vi "Initialize RF boards - with FPGA init only vi 16.3.1v7d.vi"(2 "error in":errorcluster, 3 "FPGA Interface":T1) -> (0 "error out":errorcluster, 1 "FPGA Interface 2":T1)   [LabVIEW 2012]
uses:
  openfpgaref.initrf.ctl
  <vilib>/Utility/error.llb/Error Cluster From Error Code.vi
  <vilib>/rvi/errors/niLvFpgaAdjustHostInterfaceError.vi
  <vilib>/rvi/interface/nirviReadWriteControl/nirviReadWriteControl.xnode
  FPGA Bitfiles/UHR-FleezersInst_FPGATarget_intitializeRFsyn_v1.lvbitx
  NiFpgaLv.dll
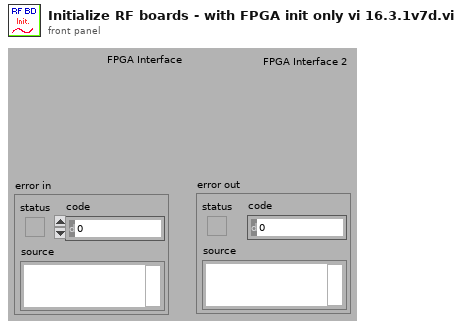
[diagram p1: front panel]
types:
  T1 = typedef "openfpgaref.initrf.ctl" = refnum<k20>
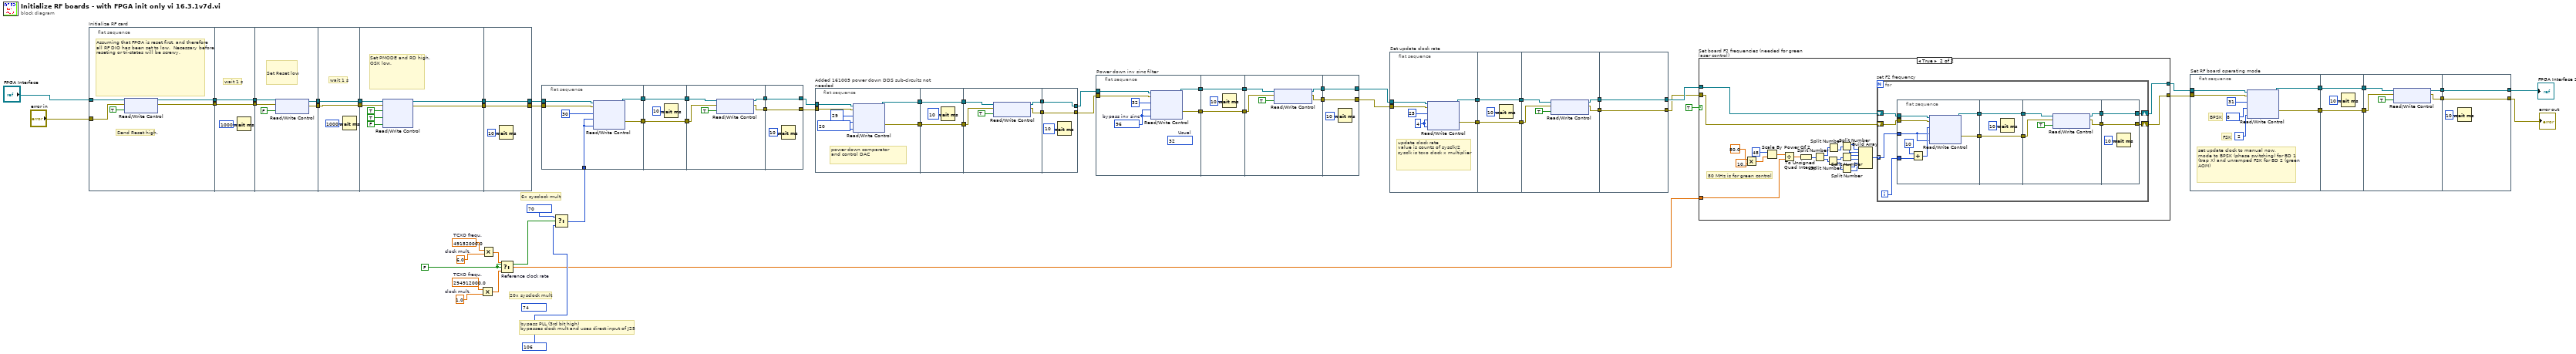
[diagram p0: block diagram]
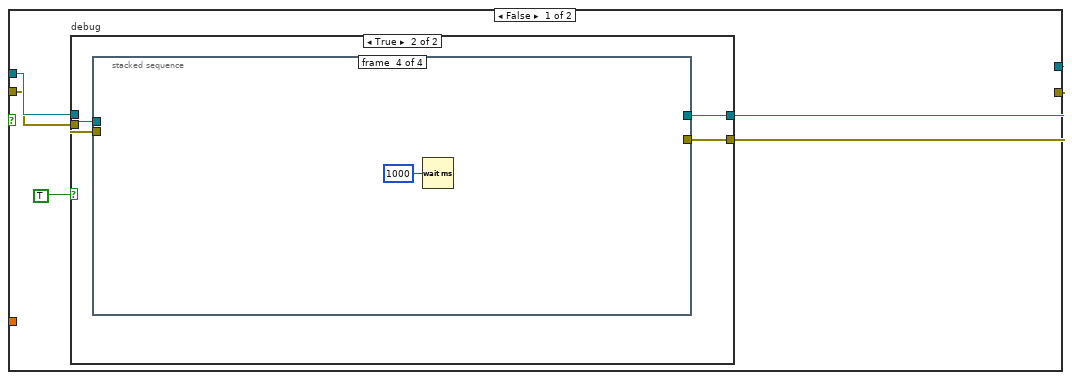
[diagram p2: hidden frame]
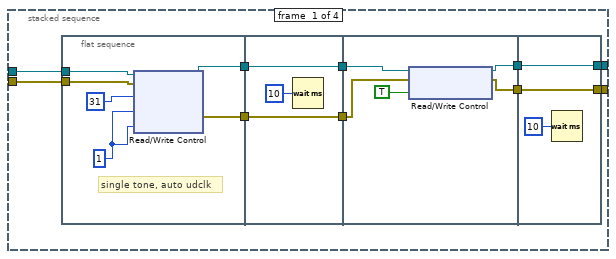
[diagram p4: hidden frame]
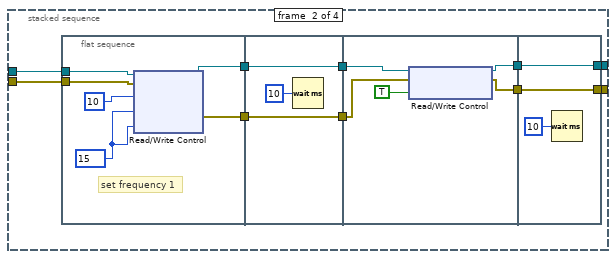
[diagram p5: hidden frame]
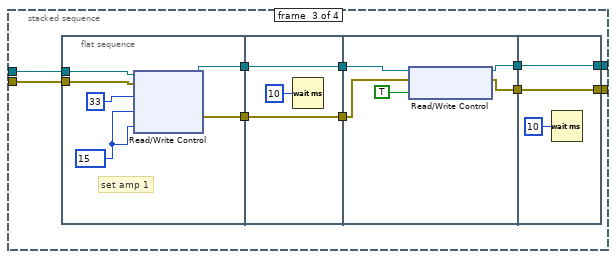
[diagram p6: hidden frame]
diagram:
  (unwired) u8 74 ("Data")
  w19 = FALSE ("s")
  w22 = 1.0  # clock mult.
  w21 = 294912000.0  # TCXO frequ.
  w25 = 6.0  # clock mult.
  w24 = 49152000.0  # TCXO frequ.
  # "bypass PLL (3rd bit high)\nbypasses clock mult and uses direct input of J25"
  # "20x sysclock mult"
  # "6x sysclock mult"
  n1 = flat-sequence "Initialize RF card" {
    tunnel: [w73] -> w68
    tunnel: [w72] -> w67
    tunnel: "error in" -> [w71]
    tunnel: "FPGA Interface" -> [w69]
    tunnel: w68 -> [w75]
    tunnel: w67 -> [w74]
    tunnel: [w75] -> w66
    tunnel: [w74] -> w65
    tunnel: w66 -> [w81]
    tunnel: w65 -> [w80]
    tunnel: [w79] -> w64
    tunnel: [w78] -> w63
    tunnel: w64 -> [w83]
    tunnel: w63 -> [w82]
    tunnel: [w83] -> w62
    tunnel: [w82] -> w61
    tunnel: w62 -> [w91]
    tunnel: w61 -> [w90]
    tunnel: [w87] -> w51
    tunnel: [w86] -> w50
    tunnel: [w93] -> w44
    tunnel: [w94] -> w45
    tunnel: w51 -> [w94]
    tunnel: w50 -> [w93]
    frame #0 {
      # "Send Reset high."
      # "Assuming that FPGA is reset first, and therefore\nall RF DIO has been set to low.  Necessary before\nreseting or tri-states will be screwy."
      n2 = xnode "Read/Write Control"("FPGA VI Reference In"=w69, "error in"=w71, "Reset Bd 1"=TRUE ("Reset")) -> ("FPGA VI Reference Out"=w73:T1, "error out"=w72:errorcluster)
    }
    frame #1 {
      # "wait 1 s"
      n3 = Wait (ms)(milliseconds to wait=u32 1000) -> ()  [unwired: 1 out]
    }
    frame #2 {
      # "Set Reset low"
      n4 = xnode "Read/Write Control"("FPGA VI Reference In"=w81, "error in"=w80, "Reset Bd 1"=FALSE ("Reset")) -> ("FPGA VI Reference Out"=w79:T1, "error out"=w78:errorcluster)
    }
    frame #3 {
      # "wait 1 s"
      n5 = Wait (ms)(milliseconds to wait=u32 1000) -> ()  [unwired: 1 out]
    }
    frame #4 {
      # "Set PMODE and RD high,\nOSK low."
      n6 = xnode "Read/Write Control"("FPGA VI Reference In"=w91, "error in"=w90, "RD"=TRUE, "PMODE"=TRUE, "OSK Bd 1"=FALSE ("OSK")) -> ("FPGA VI Reference Out"=w87:T1, "error out"=w86:errorcluster)
    }
    frame #5 {
      n7 = Wait (ms)(milliseconds to wait=u32 10) -> ()  [unwired: 1 out]
    }
  }
  n8 = Multiply(x=w21, y=w22) -> (x*y=w20:dbl)
  n9 = Multiply(x=w24, y=w25) -> (x*y=w23:dbl)
  n10 = Select "Reference clock rate"(t=w23, s=w19, f=w20) -> (s? t:f=w1:dbl)
  n11 = flat-sequence {
    tunnel: [w100] -> w60
    tunnel: [w99] -> w59
    tunnel: w45 -> [w98]
    tunnel: w44 -> [w97]
    tunnel: w17 -> [w95]
    tunnel: [w102] -> w58
    tunnel: w60 -> [w102]
    tunnel: [w101] -> w57
    tunnel: w59 -> [w101]
    tunnel: w58 -> [w108]
    tunnel: w57 -> [w107]
    tunnel: [w105] -> w49
    tunnel: [w104] -> w48
    tunnel: [w110] -> w8
    tunnel: [w111] -> w9
    tunnel: w49 -> [w111]
    tunnel: w48 -> [w110]
    frame #0 {
      n12 = xnode "Read/Write Control"("FPGA VI Reference In"=w98, "error in"=w97, "Address"=u8 30, "Data BD 1"=w95, "Data BD 2"=w95) -> ("FPGA VI Reference Out"=w100:T1, "error out"=w99:errorcluster)
    }
    frame #1 {
      n13 = Wait (ms)(milliseconds to wait=u32 10) -> ()  [unwired: 1 out]
    }
    frame #2 {
      n14 = xnode "Read/Write Control"("FPGA VI Reference In"=w108, "error in"=w107, "Update Data"=TRUE) -> ("FPGA VI Reference Out"=w105:T1, "error out"=w104:errorcluster)
    }
    frame #3 {
      n15 = Wait (ms)(milliseconds to wait=u32 10) -> ()  [unwired: 1 out]
    }
  }
  n16 = Select(t=u8 70 ("Data"), s=w19, f=u8 106 ("Data")) -> (s? t:f=w17:u8)
  n17 = flat-sequence "Added 161005 power down DDS sub-circuits not needed" {
    tunnel: [w117] -> w15
    tunnel: [w116] -> w14
    tunnel: w9 -> [w115]
    tunnel: w8 -> [w114]
    tunnel: [w119] -> w13
    tunnel: w15 -> [w119]
    tunnel: [w118] -> w12
    tunnel: w14 -> [w118]
    tunnel: w13 -> [w125]
    tunnel: w12 -> [w124]
    tunnel: [w122] -> w11
    tunnel: [w121] -> w10
    tunnel: [w128] -> w6
    tunnel: w11 -> [w126]
    tunnel: w10 -> [w128]
    tunnel: [w126] -> w7
    frame #0 {
      w112 = u8 20 ("Data")
      # "power down comparator\nand control DAC"
      n18 = xnode "Read/Write Control"("FPGA VI Reference In"=w115, "error in"=w114, "Address"=u8 29, "Data BD 1"=w112, "Data BD 2"=w112) -> ("FPGA VI Reference Out"=w117:T1, "error out"=w116:errorcluster)
    }
    frame #1 {
      n19 = Wait (ms)(milliseconds to wait=u32 10) -> ()  [unwired: 1 out]
    }
    frame #2 {
      n20 = xnode "Read/Write Control"("FPGA VI Reference In"=w125, "error in"=w124, "Update Data"=TRUE) -> ("FPGA VI Reference Out"=w122:T1, "error out"=w121:errorcluster)
    }
    frame #3 {
      n21 = Wait (ms)(milliseconds to wait=u32 10) -> ()  [unwired: 1 out]
    }
  }
  n22 = flat-sequence "Power down inv sinc filter" {
    tunnel: [w134] -> w56
    tunnel: [w133] -> w55
    tunnel: w7 -> [w132]
    tunnel: w6 -> [w131]
    tunnel: [w136] -> w54
    tunnel: w56 -> [w136]
    tunnel: [w135] -> w53
    tunnel: w55 -> [w135]
    tunnel: w54 -> [w142]
    tunnel: w53 -> [w141]
    tunnel: [w139] -> w47
    tunnel: [w138] -> w46
    tunnel: [w144] -> w36
    tunnel: [w145] -> w37
    tunnel: w47 -> [w145]
    tunnel: w46 -> [w144]
    frame #0 {
      w129 = u8 96  # bypass inv sinc
      (unwired) u8 32  # Usual
      n23 = xnode "Read/Write Control"("FPGA VI Reference In"=w132, "error in"=w131, "Address"=u8 32, "Data BD 1"=w129, "Data BD 2"=w129) -> ("FPGA VI Reference Out"=w134:T1, "error out"=w133:errorcluster)
    }
    frame #1 {
      n24 = Wait (ms)(milliseconds to wait=u32 10) -> ()  [unwired: 1 out]
    }
    frame #2 {
      n25 = xnode "Read/Write Control"("FPGA VI Reference In"=w142, "error in"=w141, "Update Data"=TRUE) -> ("FPGA VI Reference Out"=w139:T1, "error out"=w138:errorcluster)
    }
    frame #3 {
      n26 = Wait (ms)(milliseconds to wait=u32 10) -> ()  [unwired: 1 out]
    }
  }
  n27 = flat-sequence "Set update clock rate" {
    tunnel: [w151] -> w43
    tunnel: [w150] -> w42
    tunnel: w37 -> [w149]
    tunnel: w36 -> [w148]
    tunnel: [w153] -> w41
    tunnel: w43 -> [w153]
    tunnel: [w152] -> w40
    tunnel: w42 -> [w152]
    tunnel: w41 -> [w159]
    tunnel: w40 -> [w158]
    tunnel: [w156] -> w39
    tunnel: [w155] -> w38
    tunnel: [w160] -> w34
    tunnel: [w161] -> w35
    tunnel: w39 -> [w161]
    tunnel: w38 -> [w160]
    frame #0 {
      w146 = u8 4 ("Data")
      # "update clock rate\nvalue is counts of sysclk/2\nsysclk is tcxo clock x multiplier"
      n28 = xnode "Read/Write Control"("FPGA VI Reference In"=w149, "error in"=w148, "Address"=u8 25, "Data BD 1"=w146, "Data BD 2"=w146) -> ("FPGA VI Reference Out"=w151:T1, "error out"=w150:errorcluster)
    }
    frame #1 {
      n29 = Wait (ms)(milliseconds to wait=u32 10) -> ()  [unwired: 1 out]
    }
    frame #2 {
      n30 = xnode "Read/Write Control"("FPGA VI Reference In"=w159, "error in"=w158, "Update Data"=TRUE) -> ("FPGA VI Reference Out"=w156:T1, "error out"=w155:errorcluster)
    }
    frame #3 {
    }
  }
  n31 = case "Set board F2 frequencies (needed for green laser control)" shown="True" TRUE {
    tunnel: w35 -> [w166 w274]
    tunnel: w34 -> [w165 w273]
    tunnel: [w162 w271] -> w33
    tunnel: [w163 w272] -> w32
    tunnel: w1 -> [_ w251]
    frame False {
      n32 = case "debug" shown="True" TRUE {
        tunnel: w166 -> [w168 w172]
        tunnel: w165 -> [w167 w171]
        tunnel: [w168 w170] -> w163
        tunnel: [w167 w169] -> w162
        frame False {
        }
        frame True {
          n33 = stacked-sequence {
            tunnel: w172 -> [w174 w199 w226 _]
            tunnel: w171 -> [w173 w198 w225 _]
            tunnel: [_ _ w224 _] -> w170
            tunnel: [_ _ w223 _] -> w169
            frame #0 {
              n34 = flat-sequence {
                tunnel: [w186] -> w180
                tunnel: [w185] -> w179
                tunnel: w174 -> [w184]
                tunnel: w173 -> [w183]
                tunnel: [w188] -> w178
                tunnel: w180 -> [w188]
                tunnel: [w187] -> w177
                tunnel: w179 -> [w187]
                tunnel: w178 -> [w194]
                tunnel: w177 -> [w193]
                tunnel: [w191] -> w176
                tunnel: [w190] -> w175
                tunnel: [w197] -> _
                tunnel: [w195] -> _
                tunnel: w176 -> [w195]
                tunnel: w175 -> [w197]
                frame #0 {
                  w181 = u8 1 ("Data")
                  # "single tone, auto udclk"
                  n35 = xnode "Read/Write Control"("FPGA VI Reference In"=w184, "error in"=w183, "Address"=u8 31, "Data BD 1"=w181, "Data BD 2"=w181) -> ("FPGA VI Reference Out"=w186:T1, "error out"=w185:errorcluster)
                }
                frame #1 {
                  n36 = Wait (ms)(milliseconds to wait=u32 10) -> ()  [unwired: 1 out]
                }
                frame #2 {
                  n37 = xnode "Read/Write Control"("FPGA VI Reference In"=w194, "error in"=w193, "Update Data"=TRUE) -> ("FPGA VI Reference Out"=w191:T1, "error out"=w190:errorcluster)
                }
                frame #3 {
                  n38 = Wait (ms)(milliseconds to wait=u32 10) -> ()  [unwired: 1 out]
                }
              }
            }
            frame #1 {
              n39 = flat-sequence {
                tunnel: [w211] -> w205
                tunnel: [w210] -> w204
                tunnel: w199 -> [w209]
                tunnel: w198 -> [w208]
                tunnel: [w213] -> w203
                tunnel: w205 -> [w213]
                tunnel: [w212] -> w202
                tunnel: w204 -> [w212]
                tunnel: w203 -> [w219]
                tunnel: w202 -> [w218]
                tunnel: [w216] -> w201
                tunnel: [w215] -> w200
                tunnel: [w222] -> _
                tunnel: [w220] -> _
                tunnel: w201 -> [w220]
                tunnel: w200 -> [w222]
                frame #0 {
                  w206 = u8 15 ("Data")
                  # "set frequency 1"
                  n40 = xnode "Read/Write Control"("FPGA VI Reference In"=w209, "error in"=w208, "Address"=u8 10, "Data BD 1"=w206, "Data BD 2"=w206) -> ("FPGA VI Reference Out"=w211:T1, "error out"=w210:errorcluster)
                }
                frame #1 {
                  n41 = Wait (ms)(milliseconds to wait=u32 10) -> ()  [unwired: 1 out]
                }
                frame #2 {
                  n42 = xnode "Read/Write Control"("FPGA VI Reference In"=w219, "error in"=w218, "Update Data"=TRUE) -> ("FPGA VI Reference Out"=w216:T1, "error out"=w215:errorcluster)
                }
                frame #3 {
                  n43 = Wait (ms)(milliseconds to wait=u32 10) -> ()  [unwired: 1 out]
                }
              }
            }
            frame #2 {
              n44 = flat-sequence {
                tunnel: [w238] -> w232
                tunnel: [w237] -> w231
                tunnel: w226 -> [w236]
                tunnel: w225 -> [w235]
                tunnel: [w240] -> w230
                tunnel: w232 -> [w240]
                tunnel: [w239] -> w229
                tunnel: w231 -> [w239]
                tunnel: w230 -> [w246]
                tunnel: w229 -> [w245]
                tunnel: [w243] -> w228
                tunnel: [w242] -> w227
                tunnel: [w249] -> w223
                tunnel: [w247] -> w224
                tunnel: w228 -> [w247]
                tunnel: w227 -> [w249]
                frame #0 {
                  w233 = u8 15 ("Data")
                  # "set amp 1"
                  n45 = xnode "Read/Write Control"("FPGA VI Reference In"=w236, "error in"=w235, "Address"=u8 33, "Data BD 1"=w233, "Data BD 2"=w233) -> ("FPGA VI Reference Out"=w238:T1, "error out"=w237:errorcluster)
                }
                frame #1 {
                  n46 = Wait (ms)(milliseconds to wait=u32 10) -> ()  [unwired: 1 out]
                }
                frame #2 {
                  n47 = xnode "Read/Write Control"("FPGA VI Reference In"=w246, "error in"=w245, "Update Data"=TRUE) -> ("FPGA VI Reference Out"=w243:T1, "error out"=w242:errorcluster)
                }
                frame #3 {
                  n48 = Wait (ms)(milliseconds to wait=u32 10) -> ()  [unwired: 1 out]
                }
              }
            }
            frame #3 {
              n49 = Wait (ms)(milliseconds to wait=u32 1000) -> ()  [unwired: 1 out]
            }
          }
        }
      }
    }
    frame True {
      # "80 MHz is for green control"
      n50 = Multiply(x=80.0 ("Delta Frequency  (MHz)"), y=1000000.0) -> (x*y=w256:dbl)
      n51 = Scale By Power Of 2(n=48, x=w256) -> (x*2^n=w254:dbl)
      n52 = Divide(x=w254, y=w251) -> (x/y=w255:dbl)
      n53 = To Unsigned Quad Integer(1:w255) -> (0:w259:u64)
      n54 = Split Number(x=w259) -> (hi(x)=w260:u32, lo(x)=w261:u32)
      n55 = Split Number(x=w261) -> (hi(x)=w263:u16, lo(x)=w262:u16)
      n56 = Split Number(x=w260) -> (lo(x)=w264:u16)  [unwired: 1 out]
      n57 = Split Number(x=w264) -> (hi(x)=w265:u8, lo(x)=w266:u8)
      n58 = Split Number(x=w263) -> (hi(x)=w267:u8, lo(x)=w268:u8)
      n59 = Split Number(x=w262) -> (hi(x)=w269:u8, lo(x)=w270:u8)
      n60 = Build Array(w265, w266, w267, w268, w269, w270) -> (w252:u8[])
      n61 = for "set F2 frequency" {
        shift-right: [w277] -> w272
        shift-left: w274 -> [w280]
        shift-right: [w278] -> w271
        shift-left: w273 -> [w279]
        tunnel: w252 -> [w275] mode=indexing
        i -> [w276]
        n62 = flat-sequence {
          tunnel: [w294] -> w286
          tunnel: [w293] -> w285
          tunnel: w280 -> [w292]
          tunnel: w279 -> [w291]
          tunnel: w276 -> [w289]
          tunnel: w275 -> [w287]
          tunnel: [w296] -> w284
          tunnel: w286 -> [w296]
          tunnel: [w295] -> w283
          tunnel: w285 -> [w295]
          tunnel: w284 -> [w302]
          tunnel: w283 -> [w301]
          tunnel: [w299] -> w282
          tunnel: [w298] -> w281
          tunnel: [w305] -> w278
          tunnel: [w303] -> w277
          tunnel: w282 -> [w303]
          tunnel: w281 -> [w305]
          frame #0 {
            n63 = Add(x=u8 10 ("Address"), y=w289) -> (x+y=w288:i32)
            n64 = xnode "Read/Write Control"("FPGA VI Reference In"=w292, "error in"=w291, "Address"=w288, "Data BD 1"=w287, "Data BD 2"=w287) -> ("FPGA VI Reference Out"=w294:T1, "error out"=w293:errorcluster)
          }
          frame #1 {
            n65 = Wait (ms)(milliseconds to wait=u32 10) -> ()  [unwired: 1 out]
          }
          frame #2 {
            n66 = xnode "Read/Write Control"("FPGA VI Reference In"=w302, "error in"=w301, "Update Data"=TRUE) -> ("FPGA VI Reference Out"=w299:T1, "error out"=w298:errorcluster)
          }
          frame #3 {
            n67 = Wait (ms)(milliseconds to wait=u32 10) -> ()  [unwired: 1 out]
          }
        }
      }
    }
  }
  n68 = flat-sequence "Set RF board operating mode" {
    tunnel: [w312] -> w31
    tunnel: [w311] -> w30
    tunnel: w32 -> [w310]
    tunnel: w33 -> [w309]
    tunnel: [w314] -> w29
    tunnel: w31 -> [w314]
    tunnel: [w313] -> w28
    tunnel: w30 -> [w313]
    tunnel: w29 -> [w320]
    tunnel: w28 -> [w319]
    tunnel: [w317] -> w27
    tunnel: [w316] -> w4
    tunnel: [w323] -> w26
    tunnel: w27 -> [w323]
    tunnel: [w321] -> w3
    tunnel: w4 -> [w321]
    frame #0 {
      # "BPSK"
      # "FSK"
      # "set update clock to manual now,\nmode to BPSK (phase switching) for BD 1 (trap X) and unramped FSK for BD 2 (green AOM)"
      n69 = xnode "Read/Write Control"("FPGA VI Reference In"=w310, "error in"=w309, "Address"=u8 31, "Data BD 1"=u8 8 ("Data"), "Data BD 2"=u8 2 ("Data")) -> ("FPGA VI Reference Out"=w312:T1, "error out"=w311:errorcluster)
    }
    frame #1 {
      n70 = Wait (ms)(milliseconds to wait=u32 10) -> ()  [unwired: 1 out]
    }
    frame #2 {
      n71 = xnode "Read/Write Control"("FPGA VI Reference In"=w320, "error in"=w319, "Update Data"=TRUE) -> ("FPGA VI Reference Out"=w316:T1, "error out"=w317:errorcluster)
    }
    frame #3 {
      n72 = Wait (ms)(milliseconds to wait=u32 10) -> ()  [unwired: 1 out]
    }
  }
  "error out" <- w26
  "FPGA Interface 2" <- w3
